vi "Scanning Setting.vi"() -> ()   [LabVIEW 2012]
panel:
  in  "Default Z Thikness":dbl=0.15
  in  "Z Thikness":dbl=0.15
  in  "Z to Location b":dbl=410.64
  in  "Z to location a":dbl=482.42
  in  "Z to Peizo b":dbl=9.46
  in  "Z to Peizo a":dbl=11.35
  in  "Z-Offset plus":dbl=-0.45
  in  "Peizo Amp":dbl
  in  "Peizo Offset":dbl=6.0
  in  "Z Slice number":dbl=10.0
  in  "Single Line Scan":bool
  in  "Z freq":dbl=2.49875
  in  "S freq":dbl=1200.0
  in  "S-Angle Correction Z":dbl=-0.41789996905297544
  in  "S-Angle Correction S":dbl=1.4178999690529754
  in  "Z-Offset":dbl=-1.0299401197604787
  in  "S-Offset":dbl=-3.391812865497076
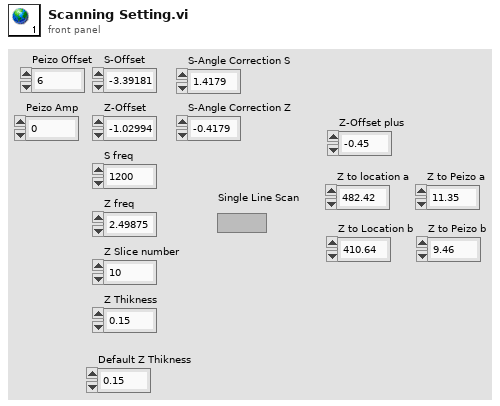
[diagram p1: front panel]
diagram:
